vi "Automated BLE_HRM.vi"() -> ()   [LabVIEW 2018]
panel:
  out "BLE_HRM":bool=TRUE
  out "Hand/Thumb":bool=TRUE
  in  "stopHRM":bool
  in  "PUL0":bool
  in  "PUL1":bool
  out "BLE Status":u32
  in  "EQF1259 com port":refnum<visa-resource-name>
  out "BLE PULSE":u32(graph)
  out "BLE_BPM":u32
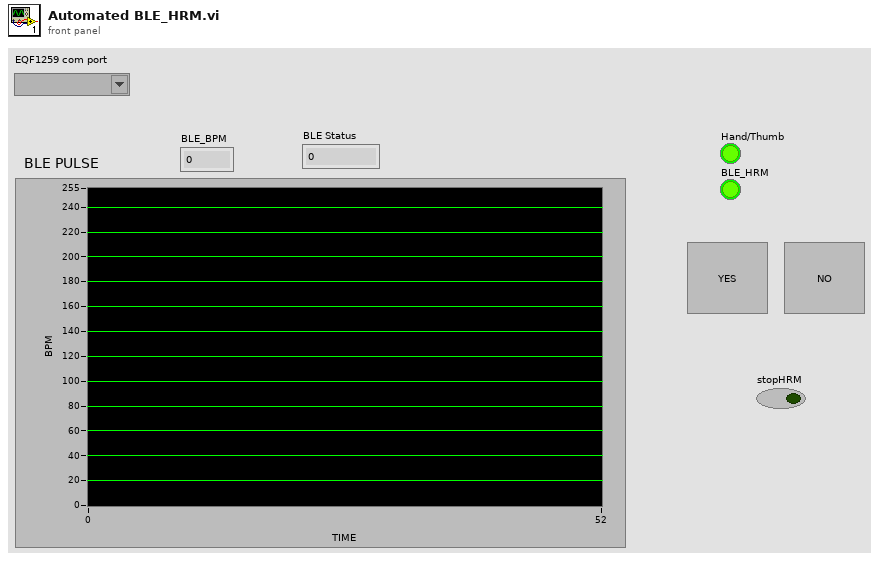
[diagram p1: front panel]
types:
  T1 = enum16{"verifyHand_Thumb", "startBLE_HRM", "readBLE_HRM", "statusBLE_HRM"}
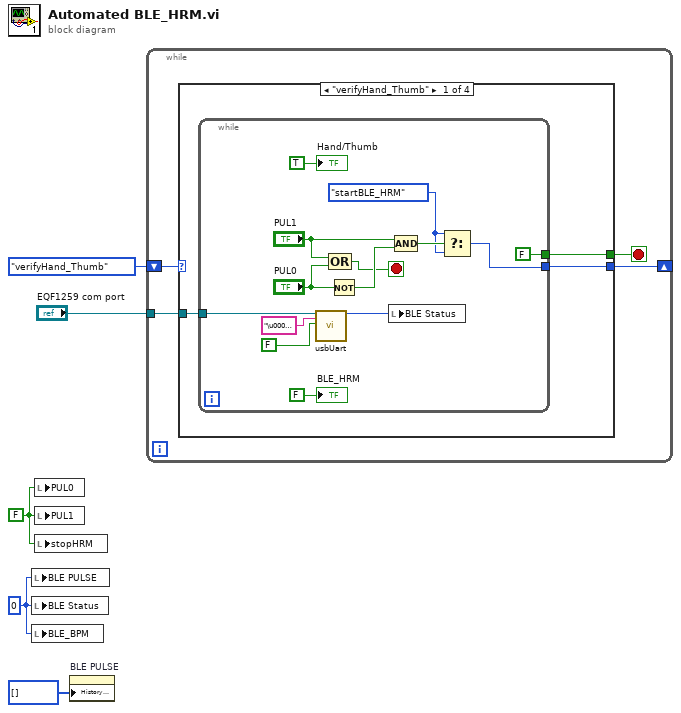
[diagram p0: block diagram]
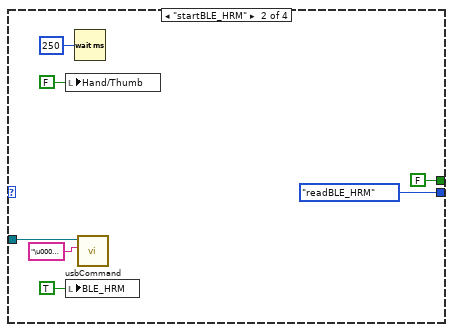
[diagram p2: hidden frame]
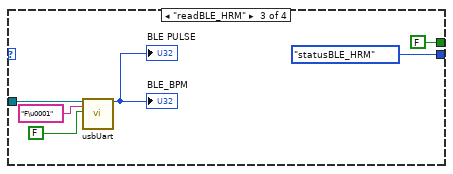
[diagram p3: hidden frame]
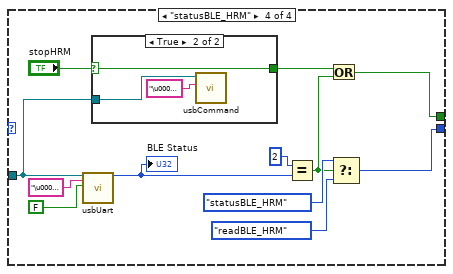
[diagram p4: hidden frame]
diagram:
  w2 = u32 0 ("BLE PULSE")
  w3 = FALSE
  n1 = local write "BLE PULSE"(w2) -> ()
  n2 = local write "BLE Status"(w2) -> ()
  n3 = local write "BLE_BPM"(w2) -> ()
  n4 = local write "PUL0"(w3) -> ()
  n5 = local write "PUL1"(w3) -> ()
  n6 = local write "stopHRM"(w3) -> ()
  n7 = property on="BLE PULSE" class="WFChart (strict)"("History Data"=u32[] []) -> ()  [unwired: 2 in, 2 out]
  n8 = while {
    tunnel: "EQF1259 com port" -> [w8]
    shift-right: [w7] -> _
    shift-left: T1."verifyHand_Thumb" -> [w9]
    stop <- w6 stop-if-true
    n9 = case shown="\"verifyHand_Thumb\"" w9 {
      tunnel: w8 -> [w10 w32 w35 w40]
      tunnel: [w12 T1."readBLE_HRM" T1."statusBLE_HRM" w47] -> w7
      tunnel: [w11 FALSE FALSE w44] -> w6
      frame "verifyHand_Thumb" {
        n10 = while {
          tunnel: [w23] -> w12
          tunnel: [FALSE] -> w11
          tunnel: w10 -> [w16]
          stop <- w20 stop-if-true
          w21 = T1."startBLE_HRM"
          n11 = call "usbUart.vi"("VISA resource name"=w16, "write buffer"="\u0002\u0001", "sdFeature"=FALSE) -> ("number[0]"=w15:u32)  [unwired: 1 in, 15 out]
          n12 = Compound Arithmetic op=OR("PUL1", "PUL0") -> (w20:bool)
          n13 = Not(x="PUL0") -> (.not. x?=w24:bool)
          n14 = local write "BLE Status"(w15) -> ()
          n15 = Compound Arithmetic op=AND("PUL1", w24) -> (w22:bool)
          n16 = Select(t=w21, s=w22, f=w21) -> (s? t:f=w23:T1)
          "Hand/Thumb" <- TRUE
          "BLE_HRM" <- FALSE
        }
      }
      frame "startBLE_HRM" {
        n17 = local write "Hand/Thumb"(FALSE) -> ()
        n18 = local write "BLE_HRM"(TRUE) -> ()
        n19 = Wait (ms)(milliseconds to wait=u32 250) -> ()  [unwired: 1 out]
        n20 = call "usbCommand.vi"("write buffer"="\u000b\u0001", "VISA resource name"=w32) -> ()  [unwired: 9 in, 1 out]
      }
      frame "readBLE_HRM" {
        n21 = call "usbUart.vi"("VISA resource name"=w35, "write buffer"="F\u0001", "sdFeature"=FALSE) -> ("number[0]"=→"BLE PULSE" →"BLE_BPM":u32)  [unwired: 1 in, 15 out]
      }
      frame "statusBLE_HRM" {
        n22 = call "usbUart.vi"("VISA resource name"=w40, "write buffer"="\u0002\u0001", "sdFeature"=FALSE) -> ("number[0]"=w51:u32)  [unwired: 1 in, 15 out]
        "BLE Status" <- w51
        n23 = case shown="True" "stopHRM" {
          selector: "stopHRM" -> [w52 w54]
          tunnel: [w52 w54] -> w41
          tunnel: w40 -> [_ w53]
          frame False {
          }
          frame True {
            n24 = call "usbCommand.vi"("write buffer"="\u000b\u0000", "VISA resource name"=w53) -> ()  [unwired: 9 in, 1 out]
          }
        }
        n25 = Equal?(x=u32 2, y=w51) -> (x = y?=w43:bool)
        n26 = Or(x=w41, y=w43) -> (x .or. y?=w44:bool)
        n27 = Select(t=T1."statusBLE_HRM", s=w43, f=T1."readBLE_HRM") -> (s? t:f=w47:T1)
      }
    }
  }
